vi "check_current_status.vi"(8 "error in (no error)":errorcluster) -> (0 "error out":errorcluster, 3 "operation to enqueue":T1)   [LabVIEW 2021]
uses:
  FGVs/AppStates.ctl
  FGVs/FGVstates.ctl
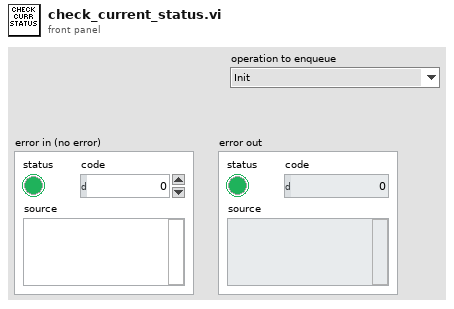
[diagram p1: front panel]
types:
  T1 = typedef "AppStates.ctl" = enum16{"Init", "Scan Music Dir", "Idle", "Playback", "Enqueue samples", "Pause playback", "Stop playback", "Exit"}
  T2 = typedef "FGVstates.ctl" = enum16{"Init", "Set", "Get", "De-Init"}
  T3 = typedef "ButtonRefs.ctl" = cluster{"Button_play":refnum<vi>, "Button_pause":refnum<vi>, "Button_stop":refnum<vi>, "Playback status":refnum<vi>, "Playback Timeline":refnum<vi>, "Right Channel":refnum<vi>, "Left Channel":refnum<vi>, "Skip Forward Button":refnum<vi>, "Skip Back Button":refnum<vi>, "Playlist":refnum<vi>}
  T4 = typedef "playback status.ctl" = enum16{"playback", "pause", "stop"}
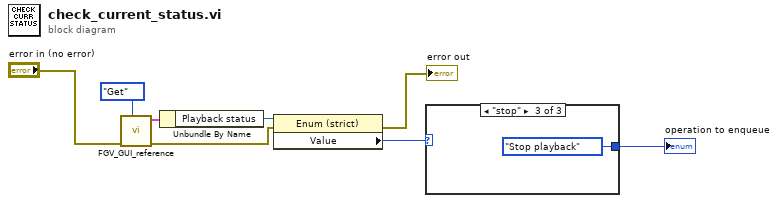
[diagram p0: block diagram]
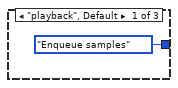
[diagram p2: hidden frame]
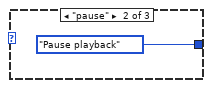
[diagram p3: hidden frame]
diagram:
  n1 = call "FGV_GUI_reference.vi"("FGV states"=FGVstates."Get", "error in (no error)"="error in (no error)") -> ("error out"=w2:errorcluster, "Button refs Out"=w5:T3)  [unwired: 8 in]
  n2 = Unbundle By Name(w5) -> ("Playback status"=w6:refnum<vi>)
  n3 = property class="Enum (strict)"(reference=w6, error in=w2) -> (error out=→"error out":errorcluster, "Value"=w7:T4)  [unwired: 1 out]
  n4 = case shown="\"stop\"" w7 {
    tunnel: [AppStates."Enqueue samples" ("element") AppStates."Pause playback" ("element") AppStates."Stop playback" ("element")] -> w8
    frame "playback", Default {
    }
    frame "pause" {
    }
    frame "stop" {
    }
  }
  "operation to enqueue" <- w8
